vi "SetImageBufferSize.vi"(8 "error in (no error)":errorcluster, 10 "max queue size (-1, unlimited)":i32, 11 "Camera in":refnum<class "Camera.lvclass">) -> (0 "error out":errorcluster, 3 "Camera out":refnum<class "Camera.lvclass">)   [LabVIEW 2020, in "Camera.lvlib" / "Camera.lvclass"]
uses:
  Camera.lvclass
  Camera.lvclass/Camera.ctl
  <vilib>/vision/Image Controls.llb/IMAQ Image.ctl
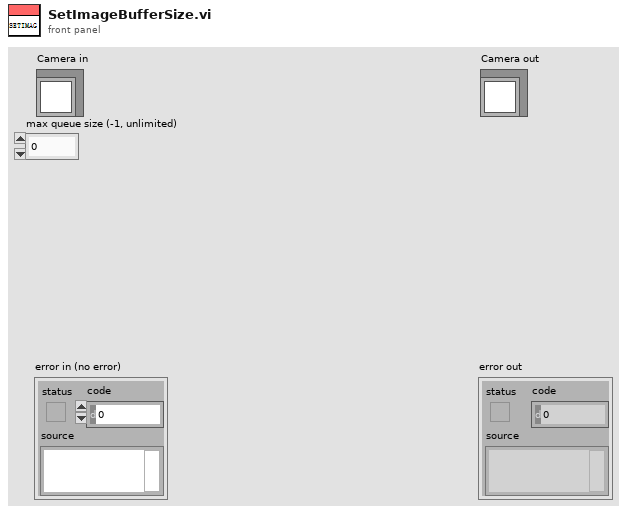
[diagram p1: front panel]
types:
  T1 = typedef "IMAQ Image.ctl" = refnum<image>
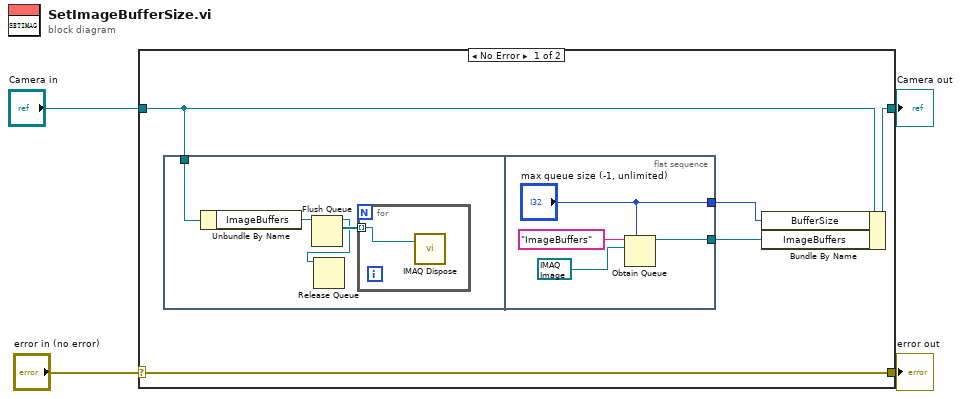
[diagram p0: block diagram]
diagram:
  n1 = case shown="No Error" "error in (no error)" {
    selector: "error in (no error)" -> [w9 w20]
    tunnel: [w9 w20] -> w3
    tunnel: [w7 w19] -> w1
    tunnel: "Camera in" -> [w8 w19]
    frame No Error {
      n2 = flat-sequence {
        tunnel: w8 -> [w13]
        tunnel: [w16] -> w6
        tunnel: ["max queue size (-1, unlimited)"] -> w5
        frame #0 {
          n3 = Unbundle By Name(w13) -> ("ImageBuffers"=w12:refnum<queue>)
          n4 = Flush Queue(queue=w12) -> (queue out=w10:refnum<queue>, remaining elements=w11:T1[])  [unwired: 1 in, 1 out]
          n5 = Release Queue(queue=w10) -> ()  [unwired: 2 in, 3 out]
          n6 = for {
            tunnel: w11 -> [w14] mode=indexing
            n7 = call "IMAQ Dispose"("Image"=w14) -> ()  [unwired: 5 in, 1 out]
          }
        }
        frame #1 {
          n8 = Obtain Queue(max queue size (-1, unlimited)="max queue size (-1, unlimited)", name (unnamed)="ImageBuffers", element data type=T1 refnum ("New Image")) -> (queue out=w16:refnum<queue>)  [unwired: 2 in, 2 out]
        }
      }
      n9 = Bundle By Name(cluster=w8, "BufferSize"=w5, "ImageBuffers"=w6) -> (w7:refnum<class "Camera.lvclass">)
    }
    frame Error {
    }
  }
  "error out" <- w3
  "Camera out" <- w1
